vi "DIALOG BOX HFRR ADV.vi"(1 "Status":string="Warning:\nTrained and authorized users only! \nEnsure all positioners are tightened and specimens are mounted securely.\nMoving machinery can cause serious injuries - keep away when equipment is in operation. \n", 3 "error in":errorcluster) -> (8 "Continue":bool, 9 "Cancel":bool, 10 "error out":errorcluster)   [LabVIEW 2025]
uses:
  <vilib>/Utility/traverseref.llb/VI Scripting - Traverse.lvlib
  <vilib>/Utility/traverseref.llb/TRef TravTarget.ctl
panel:
  in  "Cancel":bool
  in  "Boolean":bool
  in  "Continue":bool
  # "Service Mode"
  # "CAUTION - Improper use of Service Mode could result in loss of Machine Operation, permanent Machine damage, or serious personal Injury."
  # "Service Mode is intended for qualified professionals to conduct diagnostics, repairs, \nand maintenance on HFRR ADV in a controlled and safe workshop environment.\n\nWhen working on a machine or using Service Mode always refer to the Manual for safety \nprecautions and procedures, and always adhere to industry best practices.\n\nVisit https://www.paltro.com/contact-forms/contact-customer-support for more information"
  # "Warning:\nTrained and authorized users only! Ensure all positioners are tightened and specimens are mounted securely.\nMoving machinery can cause serious injuries - keep away when equipment is in operation."
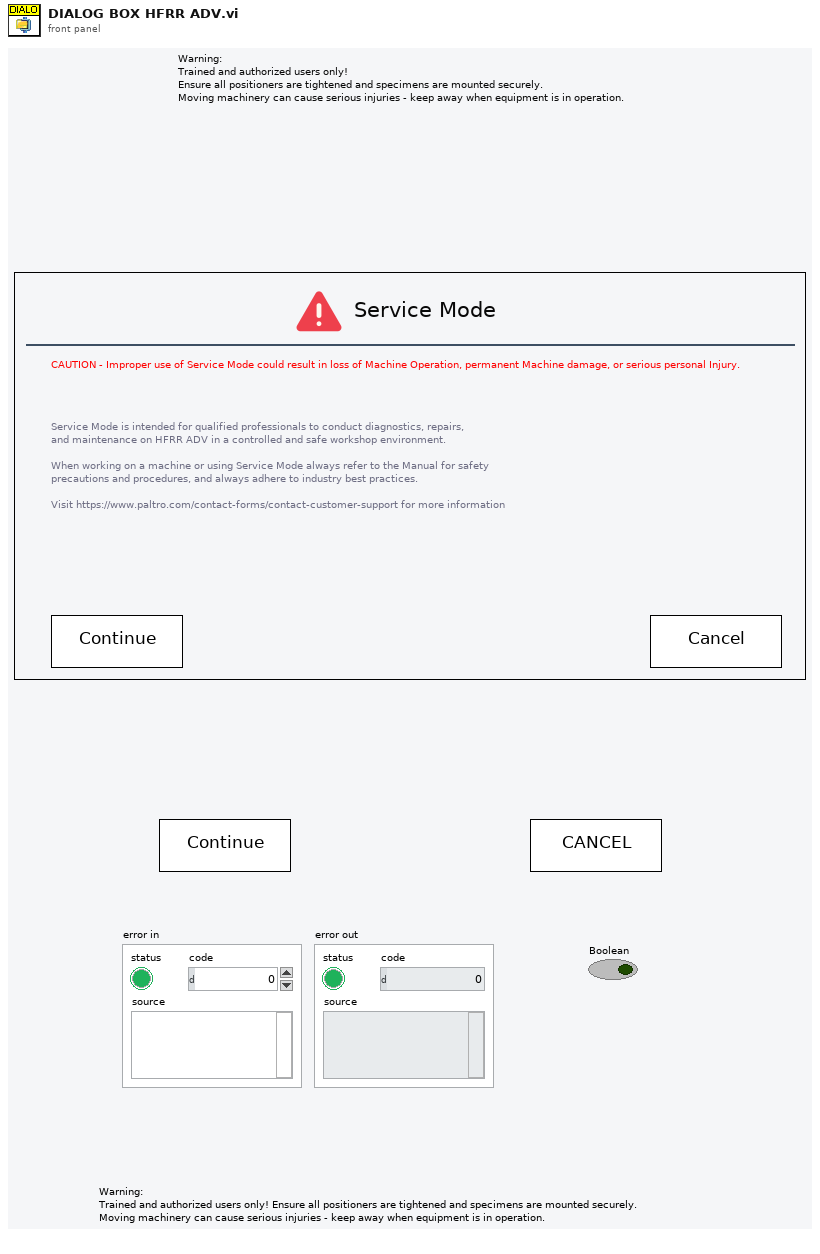
[diagram p1: front panel]
types:
  T1 = typedef "TRef TravTarget.ctl" = enum16{"FP", "BD", "Other"}
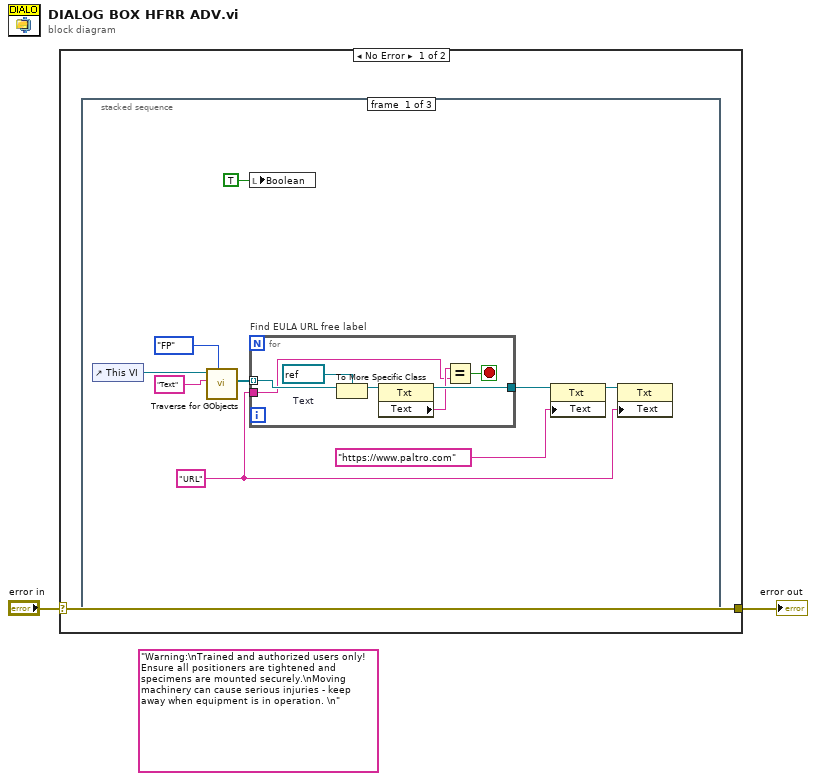
[diagram p0: block diagram]
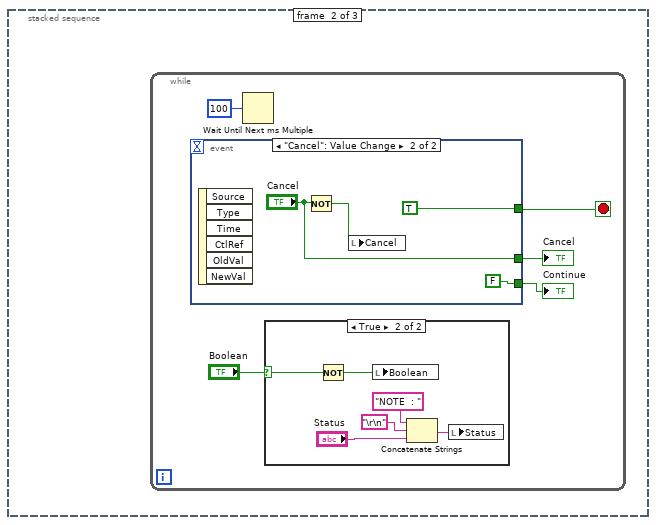
[diagram p2: hidden frame]
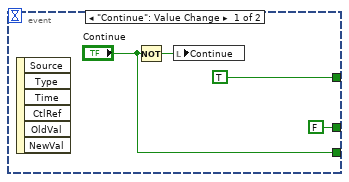
[diagram p4: hidden frame]
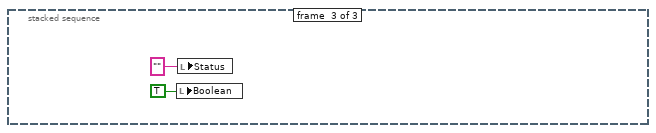
[diagram p5: hidden frame]
diagram:
  (unwired) "Warning:\nTrained and authorized users only! Ensure all positioners are tightened and specimens are mounted securely.\nMoving machinery can cause serious injuries - keep away when equipment is in operation. \n" ("message")
  n1 = case shown="No Error" "error in" {
    selector: "error in" -> [w3 _]
    tunnel: [w3 _] -> w1
    frame No Error {
      n2 = stacked-sequence {
        frame #0 {
          w10 = "URL"
          n3 = control-ref of="This VI"() -> (w7:refnum<vi>)
          n4 = call <vilib>:"Traverse for GObjects.vi"("Traverse Target"=TRef_TravTarget."FP", "Class Name"="Text", "VI Refnum"=w7) -> ("References"=w5:refnum<vi>[])  [unwired: 5 in, 3 out]
          n5 = local write "Boolean"(TRUE ("Boolean")) -> ()
          n6 = for "Find EULA URL free label" {
            tunnel: w5 -> [w19] mode=indexing
            tunnel: [w16] -> w4
            tunnel: w10 -> [w14]
            stop <- w13 stop-if-true
            w18 = refnum<vi> refnum  # Text
            n7 = To More Specific Class(target class=w18, reference=w19) -> (specific class reference=w17:refnum<vi>)  [unwired: 1 in, 1 out]
            n8 = property class="Txt"(reference=w17) -> (reference out=w16:refnum<vi>, "Text"=w15:string)  [unwired: 1 in, 1 out]
            n9 = Equal?(x=w15, y=w14) -> (x = y?=w13:bool)
          }
          n10 = property class="Txt"(reference=w4, "Text"="https://www.paltro.com") -> (reference out=w9:refnum<vi>)  [unwired: 1 in, 1 out]
          n11 = property class="Txt"(reference=w9, "Text"=w10) -> ()  [unwired: 1 in, 2 out]
        }
        frame #1 {
          n12 = while {
            stop <- w23 stop-if-true
            n13 = event shown="[1] \"Cancel\": Value Change" {
              selector: _ -> [_ _]
              dyn-events: _ -> [_ _]
              timeout: _ -> [_ _]
              tunnel: [TRUE TRUE] -> w23
              tunnel: [FALSE ("Skip") "Cancel"] -> w21
              tunnel: ["Continue" FALSE] -> w20
              event "Continue": Value Change {
                n14 = event-data() -> ()  [unwired: 1 in, 6 out]
                n15 = Not(x="Continue") -> (.not. x?=w33:bool)
                n16 = local write "Continue"(w33) -> ()
              }
              event "Cancel": Value Change {
                n17 = event-data() -> ()  [unwired: 1 in, 6 out]
                n18 = Not(x="Cancel") -> (.not. x?=w37:bool)
                n19 = local write "Cancel"(w37) -> ()
              }
            }
            "Cancel" <- w21
            "Continue" <- w20
            n20 = Wait Until Next ms Multiple(millisecond multiple=100) -> ()  [unwired: 1 out]
            n21 = case shown="True" "Boolean" {
              selector: "Boolean" -> [_ w29]
              frame False {
              }
              frame True {
                n22 = Not(x=w29) -> (.not. x?=w28:bool)
                n23 = local write "Boolean"(w28) -> ()
                n24 = Concatenate Strings("NOTE  : ", "\r\n", "Status") -> (w27:string)
                n25 = local write "Status"(w27) -> ()
              }
            }
          }
        }
        frame #2 {
          n26 = local write "Boolean"(TRUE ("Boolean")) -> ()
          n27 = local write "Status"("") -> ()
        }
      }
    }
    frame Error {
    }
  }
  "error out" <- w1
